vi "FTP Worker RD v1.0.vi"(8 "error in (no error)":errorcluster, 11 "Enable FTP?":bool) -> (0 "error out":errorcluster)   [LabVIEW 2019]
doc: "Uploads a specified file to an FTP server based on preferences set in the Configurator. \n\nNOTE: FTP is insecure and it is recommended to use AWS S3 instead. MODAQ is written in LabVIEW 2019 and this version has no native SFTP support. \n\n2020 NREL"
uses:
  Globals and Definitions/Initialization Globals.vi
  Globals and Definitions/RT Globals RD v1.0.vi
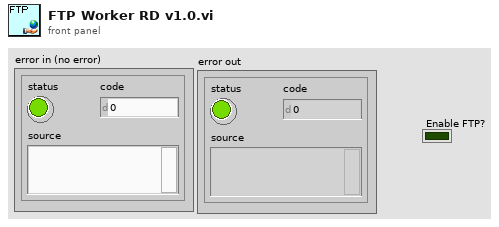
[diagram p1: front panel]
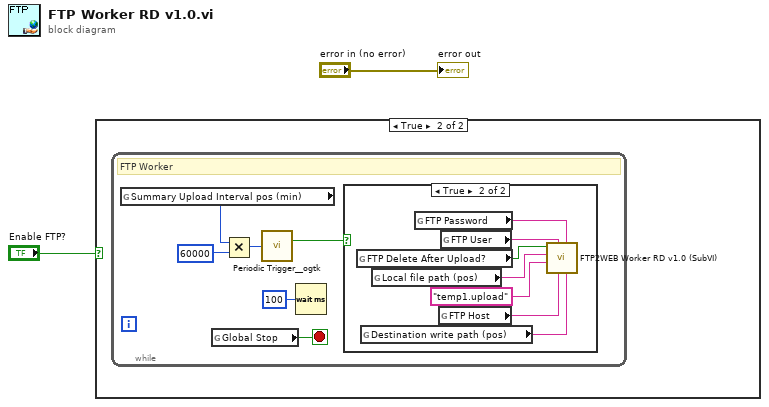
[diagram p0: block diagram]
diagram:
  n1 = case shown="True" "Enable FTP?" {
    frame False {
    }
    frame True {
      n2 = while {
        stop <- w4 stop-if-true
        # "FTP Worker"
        n3 = global read "Initialization Globals.vi" "Summary Upload Interval pos (min)"() -> (w5:i32)
        n4 = global read "RT Globals RD v1.0.vi" "Global Stop"() -> (w4:bool)
        n5 = Multiply(x=w5, y=60000) -> (x*y=w7:i32)
        n6 = call <userlib>:"Periodic Trigger__ogtk.vi"("time (ms)"=w7) -> ("Triggered"=w3:bool)  [unwired: 12 in, 2 out]
        n7 = Wait (ms)(milliseconds to wait=u32 100) -> ()  [unwired: 1 out]
        n8 = case shown="True" w3 {
          frame False {
          }
          frame True {
            n9 = global read "Initialization Globals.vi" "FTP Delete After Upload?"() -> (w13:bool)
            n10 = global read "Initialization Globals.vi" "Destination write path (pos)"() -> (w9:string)
            n11 = global read "Initialization Globals.vi" "Local file path (pos)"() -> (w12:string)
            n12 = global read "Initialization Globals.vi" "FTP Password"() -> (w15:string)
            n13 = global read "Initialization Globals.vi" "FTP Host"() -> (w10:string)
            n14 = global read "Initialization Globals.vi" "FTP User"() -> (w14:string)
            n15 = call "FTP2WEB Worker RD v1.0 (SubVI).vi"("FTP Remote Path"=w9, "FTP Password"=w15, "FTP Host"=w10, "FTP Username"=w14, "Temp Filename"="temp1.upload" ("name or relative path"), "Local File Path"=w12, "FTP Delete After Upload?"=w13) -> ()  [unwired: 4 in, 1 out]
          }
        }
      }
    }
  }
  "error out" <- "error in (no error)"
